vi "Serialize Configuration.vi"(8 "error in (no error)":errorcluster, 11 "Configuration":T1) -> (0 "error out":errorcluster, 3 "Serialized Configuration":string)   [LabVIEW 2020, in "ADAS PE Template.lvlib" / "ADAS PE Template.lvclass"]
uses:
  ADAS PE Template.lvclass
  Configuration.ctl
  <vilib>/ADAS Record/Utilities/ADAS Utilities.lvlib
panel:
  # "#via_ignore"
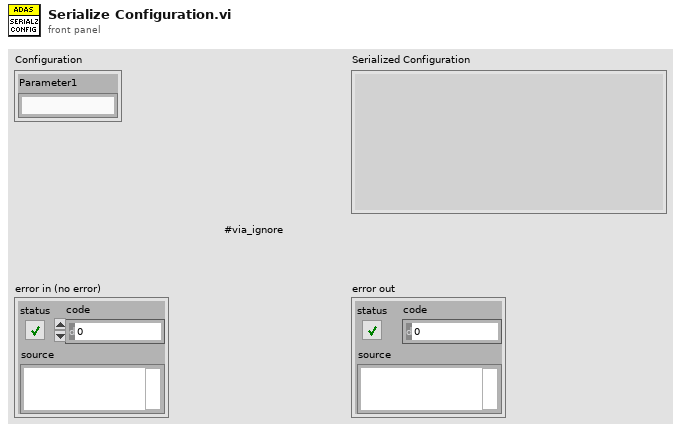
[diagram p1: front panel]
types:
  T1 = typedef "ADAS PE Template.lvlib/ADAS PE Template.lvclass/Configuration.ctl" = cluster{"Parameter1":string}
  T2 = typedef "ADAS Utilities.lvlib/Config Version.ctl" = cluster{"Major":u32, "Minor":u32, "Fix":u32, "Build":u32}
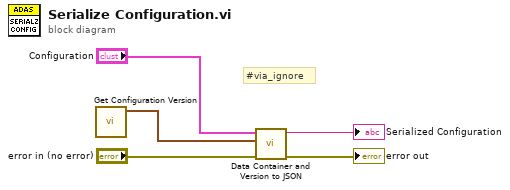
[diagram p0: block diagram]
diagram:
  # "#via_ignore"
  n1 = call "Get Configuration Version.vi"() -> ("Version"=w3:T2)  [unwired: 11 in]
  n2 = call <vilib>:"Data Container and Version to JSON.vi"("error in (no error)"="error in (no error)", "Version"=w3, "Container Variant"="Configuration") -> ("error out"=→"error out":errorcluster, "JSON string"=→"Serialized Configuration":string)  [unwired: 7 in]
